vi "GE 5565PIORC.DMA.Configure.vi"(7 "transfer direction":enum16{"Host to RFM", "RFM to Host"}(ring), 8 "error in (no error)":errorcluster, 9 "transfer size (-1: all)":i32=-1, 10 "DMA Transfer Spec":T1 {"Block Descriptors"."descriptor params"."data ptr (lower)" format="%.0x"; "Block Descriptors"."descriptor params"."data ptr (upper)" format="%.0x"; "Block Descriptors"."descriptor params"."data size" format="%.0x"; "Block Descriptors"."descriptor params"."next descriptor ptr" format="%.0x"; "Block Descriptors"."descriptor size" format="%08x"; "Block Descriptors"."descriptor ptr (RFM)" format="%08x"; "Block Descriptors"."descriptor ptr (VISA)" format="%08x"; "RFM offset" format="%08x"}, 11 "GE 5565PIORC in":refnum<class "GE 5565PIORC.lvclass">) -> (0 "error out":errorcluster, 3 "GE 5565PIORC out":refnum<class "GE 5565PIORC.lvclass">)   [LabVIEW 2024, in "GE 5565PIORC.lvclass"]
doc: "Configures the required registers on the GE 5565PIORC to prepare for a DMA transfer as defined by <B>DMA Transfer Spec</B> and for the specified <B>transfer direction</B>. The <b>transfer size</b> can be used to transfer a subset of the <b>DMA Transfer Spec</b>, and is specfied in bytes."
uses:
  GE 5565PIORC.lvclass
  Typedefs/GE 5565PIORC.Typedef.DMA Transfer Spec.ctl
  Typedefs/GE 5565PIORC.Typedef.DMA Block Descriptor.ctl
  Typedefs/GE 5565PIORC.Typedef.DMA Block Descriptor Params.ctl
  GE 5565PIORC.lvclass/GE 5565PIORC.ctl
  GE 5565PIORC.DMA.Get Transfer Components (Scatter-Gather).vi
  Properties/Registers/GE 5565PIORC.Registers.Local Configuration.Read.vi
  Properties/Registers/GE 5565PIORC.Registers.Local Configuration.Read (U32).vi
  Properties/Registers/GE 5565PIORC.Registers.Local Configuration.Write.vi
  Properties/Registers/GE 5565PIORC.Registers.Local Configuration.Write (U32).vi
  GE 5565PIORC.Bit Manipulation.Set Bit.vi
  GE 5565PIORC.Bit Manipulation.Set Bit (U32).vi
  GE 5565PIORC.DMA.Scatter-Gather.Set Descriptor Params.vi
  GE 5565PIORC.Registers.Read.vi
  GE 5565PIORC.Registers.Read (U32).vi
  GE 5565PIORC.Registers.Write.vi
  GE 5565PIORC.Registers.Write (U32).vi
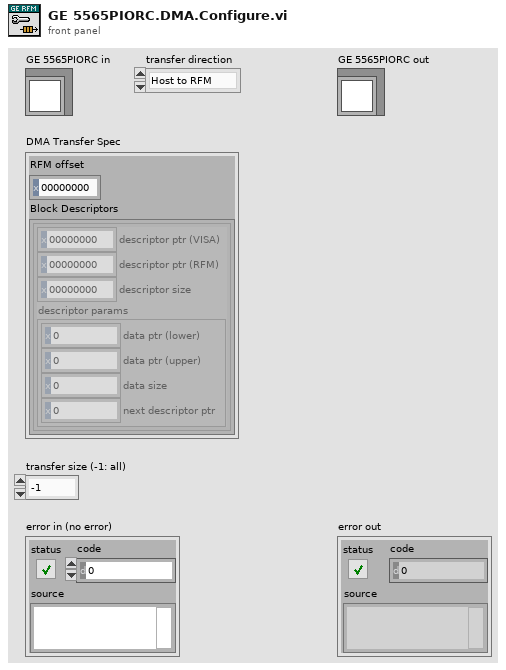
[diagram p1: front panel]
types:
  T1 = typedef "GE 5565PIORC.lvclass/GE 5565PIORC.Typedef.DMA Transfer Spec.ctl" = cluster{"RFM offset":u32, "Block Descriptors":T2[]}
  T2 = typedef "GE 5565PIORC.lvclass/GE 5565PIORC.Typedef.DMA Block Descriptor.ctl" = cluster{"descriptor ptr (VISA)":u32, "descriptor ptr (RFM)":u32, "descriptor size":u32, "descriptor params":T3}
  T3 = typedef "GE 5565PIORC.lvclass/GE 5565PIORC.Typedef.DMA Block Descriptor Params.ctl" = cluster{"data ptr (lower)":u32, "data ptr (upper)":u32, "data size":u32, "next descriptor ptr":u32}
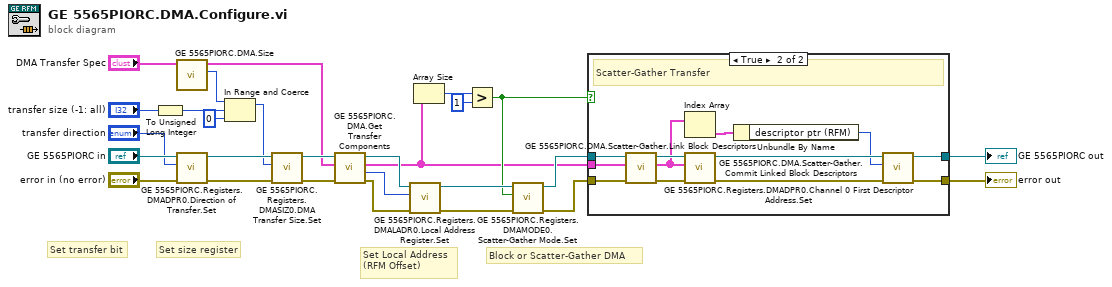
[diagram p0: block diagram]
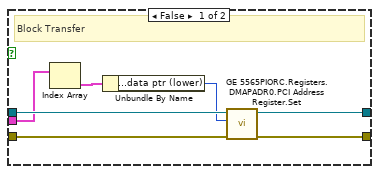
[diagram p2: hidden frame]
diagram:
  # "Block or Scatter-Gather DMA"
  # "Set Local Address (RFM Offset)"
  # "Set size register"
  # "Set transfer bit"
  n1 = To Unsigned Long Integer(number="transfer size (-1: all)") -> (unsigned 32bit integer=w3:u32)
  n2 = call "GE 5565PIORC.DMA.Size.vi"("DMA Transfer Spec"="DMA Transfer Spec") -> ("transfer size (bytes)"=w4:u32, "DMA Transfer Spec dup"=w7:T1)  [unwired: 9 in]
  n3 = call "GE 5565PIORC.Registers.DMADPR0.Direction of Transfer.Set.vi"("error in (no error)"="error in (no error)", "Transfer Direction"="transfer direction", "GE 5565PIORC in"="GE 5565PIORC in") -> ("error out"=w24:errorcluster, "GE 5565PIORC out"=w25:refnum<class "GE 5565PIORC.lvclass">)  [unwired: 7 in]
  n4 = In Range and Coerce(upper limit=w4, x=w3, lower limit=u32 0) -> (coerced(x)=w1:u32)  [unwired: 1 out]
  n5 = call "GE 5565PIORC.Registers.DMASIZ0.DMA Transfer Size.Set.vi"("error in (no error)"=w24, "DMA Transfer Size (Bytes)"=w1, "GE 5565PIORC in"=w25) -> ("error out"=w11:errorcluster, "GE 5565PIORC out"=w12:refnum<class "GE 5565PIORC.lvclass">)  [unwired: 7 in]
  n6 = call-poly "GE 5565PIORC.DMA.Get Transfer Components.vi"("error in (no error)"=w11, "DMA Transfer Spec in"=w7, "GE 5565PIORC in"=w12) -> ("error out"=w9:errorcluster, "RFM offset"=w6:u32, "Block Descriptors"=w8:T2[], "GE 5565PIORC out"=w10:refnum<class "GE 5565PIORC.lvclass">)  [unwired: 5 in]
  n7 = call "GE 5565PIORC.Registers.DMALADR0.Local Address Register.Set.vi"("error in (no error)"=w9, "Local Address Register"=w6, "GE 5565PIORC in"=w10) -> ("error out"=w22:errorcluster, "GE 5565PIORC out"=w21:refnum<class "GE 5565PIORC.lvclass">)  [unwired: 7 in]
  n8 = Array Size(array=w8) -> (size(s)=w20:i32)
  n9 = Greater?(x=w20, y=1) -> (0:w18:bool)
  n10 = call "GE 5565PIORC.Registers.DMAMODE0.Scatter-Gather Mode.Set.vi"("error in (no error)"=w22, "Scatter-Gather Mode"=w18, "GE 5565PIORC in"=w21) -> ("error out"=w16:errorcluster, "GE 5565PIORC out"=w17:refnum<class "GE 5565PIORC.lvclass">)  [unwired: 7 in]
  n11 = case shown="True" w18 {
    tunnel: w8 -> [w28 w36]
    tunnel: w17 -> [w33 w40]
    tunnel: w16 -> [w32 w38]
    tunnel: [w30 w43] -> w15
    tunnel: [w29 w42] -> w14
    frame False {
      # "Block Transfer"
      n12 = Index Array(array=w28) -> (element=w34:T2)  [unwired: 1 in]
      n13 = Unbundle By Name(w34) -> ("descriptor params.data ptr (lower)"=w31:u32)
      n14 = call "GE 5565PIORC.Registers.DMAPADR0.PCI Address Register.Set.vi"("error in (no error)"=w32, "PCI Address Register"=w31, "GE 5565PIORC in"=w33) -> ("error out"=w29:errorcluster, "GE 5565PIORC out"=w30:refnum<class "GE 5565PIORC.lvclass">)  [unwired: 7 in]
    }
    frame True {
      # "Scatter-Gather Transfer"
      n15 = call "GE 5565PIORC.DMA.Scatter-Gather.Link Block Descriptors.vi"("error in (no error)"=w38, "Block Descriptors"=w36, "GE 5565PIORC in"=w40) -> ("error out"=w37:errorcluster, "Linked Block Descriptors"=w35:T2[], "GE 5565PIORC out"=w39:refnum<class "GE 5565PIORC.lvclass">)  [unwired: 6 in]
      n16 = Index Array(array=w35) -> (element=w46:T2)  [unwired: 1 in]
      n17 = call "GE 5565PIORC.DMA.Scatter-Gather.Commit Linked Block Descriptors.vi"("error in (no error)"=w37, "Linked Block Descriptors"=w35, "GE 5565PIORC in"=w39) -> ("error out"=w45:errorcluster, "GE 5565PIORC out"=w44:refnum<class "GE 5565PIORC.lvclass">)  [unwired: 7 in]
      n18 = Unbundle By Name(w46) -> ("descriptor ptr (RFM)"=w41:u32)
      n19 = call "GE 5565PIORC.Registers.DMADPR0.Channel 0 First Descriptor Address.Set.vi"("error in (no error)"=w45, "Channel 0 First Descriptor Address"=w41, "GE 5565PIORC in"=w44) -> ("error out"=w42:errorcluster, "GE 5565PIORC out"=w43:refnum<class "GE 5565PIORC.lvclass">)  [unwired: 7 in]
    }
  }
  "GE 5565PIORC out" <- w15
  "error out" <- w14
